vi "Lokomat MVIC EMG Processing SubVI.vi"(2 "EMG Channel":i32, 3 "Post-process":u16(ring)=1 items=["RAW EMG", "Linear Envelope"], 4 "Input Array":sgl[][](array[numeric]), 5 "Do Not Remove Baseline":bool=TRUE) -> (0 "EMG Max":dbl, 1 "EMG":dbl[](graph))   [LabVIEW 2011]
uses:
  <vilib>/Analysis/NI_AALBase.lvlib
  <vilib>/Analysis/baseanly.llb/Mean (DBL).vi
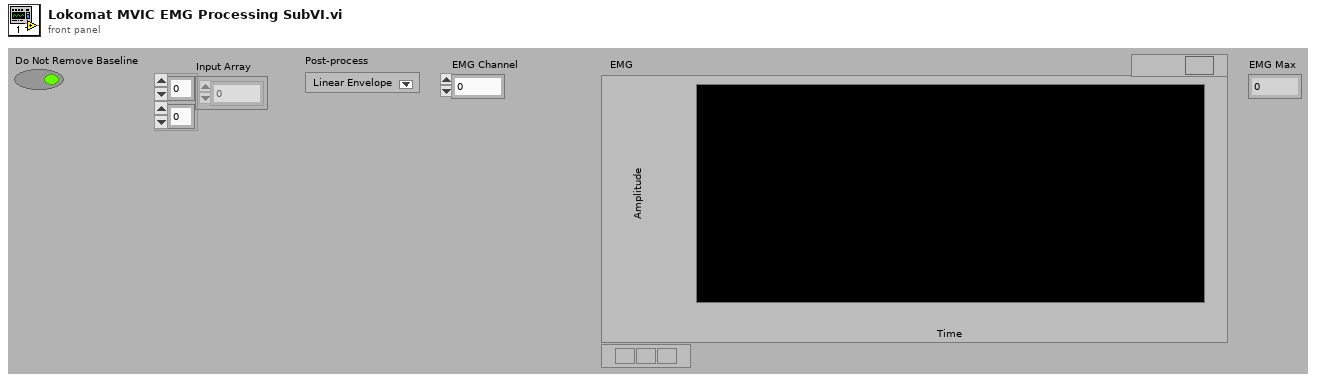
[diagram p1: front panel]
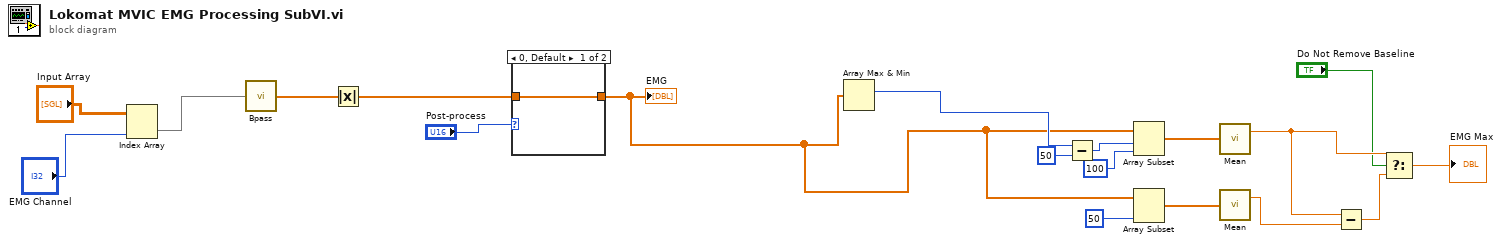
[diagram p0: block diagram]
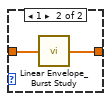
[diagram p2: hidden frame]
diagram:
  n1 = Index Array(array="Input Array", index (col)="EMG Channel") -> (element=w11:sgl[])  [unwired: 1 in]
  n2 = call "Bpass.vi"("Input Array"=w11) -> ("Output Array"=w2:dbl[])
  n3 = Absolute Value(x=w2) -> (abs(x)=w1:dbl[])
  n4 = case shown="0, Default" "Post-process" {
    tunnel: w1 -> [w20 w22]
    tunnel: [w20 w21] -> w10
    frame 0, Default {
    }
    frame 1 {
      n5 = call "Linear Envelope_Burst Study.vi"("Signals"=w22) -> ("Filtered Signals"=w21:dbl[])
    }
  }
  "EMG" <- w10
  n6 = Array Max & Min(array=w10) -> (max index (indices)=w13:i32)  [unwired: 3 out]
  n7 = Subtract(x=w13, y=50) -> (x-y=w15:i32)
  n8 = Array Subset(array=w10, index=w15, length=100) -> (w12:dbl[])
  n9 = Array Subset(array=w10, length=50) -> (w8:dbl[])  [unwired: 1 in]
  n10 = call-poly <vilib>:"Mean.vi"("X"=w12) -> ("mean"=w7:dbl)  [unwired: 1 out]
  n11 = call-poly <vilib>:"Mean.vi"("X"=w8) -> ("mean"=w6:dbl)  [unwired: 1 out]
  n12 = Subtract(x=w7, y=w6) -> (x-y=w5:dbl)
  n13 = Select(t=w7, s="Do Not Remove Baseline", f=w5) -> (s? t:f=→"EMG Max":dbl)
